vi "Process metadata.vi"(0 "reference in":refnum<class "Force Curve_tdms.lvclass">, 5 "error in (no error)":errorcluster) -> (14 "reference out":refnum<class "Force Curve_tdms.lvclass">, 19 "error out":errorcluster)   [LabVIEW 2019, in "Force Curve_tdms.lvclass"]
uses:
  Force Curve_tdms.lvclass
  TDMS_DataHandler_class/property name combo box.ctl
  Fcurve Meta data analysis.ctl
  TDMS_DataHandler_class/TDMS_DataHandler.lvclass
panel:
  out "Fcurve Raw Metadata.property names":string[](array[string])
  out "Fcurve Raw Metadata.property values":variant[](array[variant])
  out "Array":i32[](array[numeric])
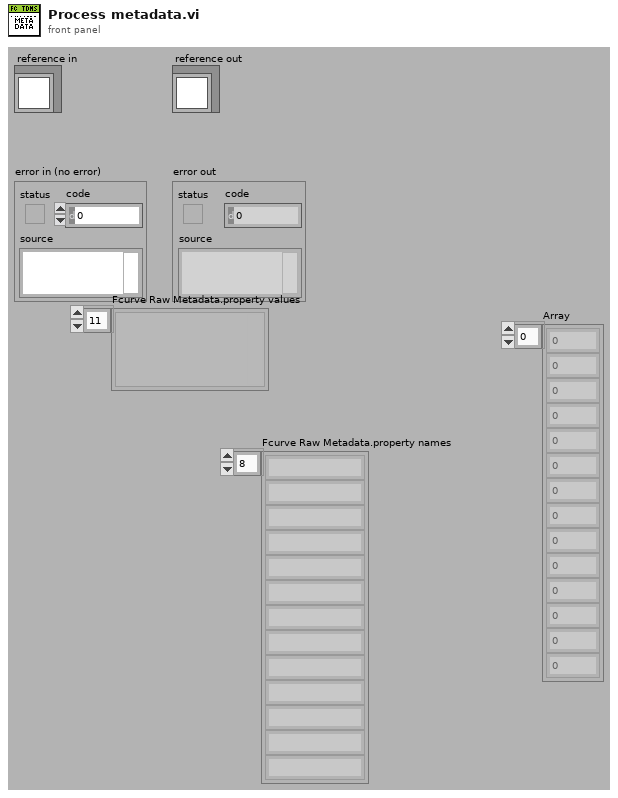
[diagram p1: front panel]
types:
  T1 = typedef "TDMS_DataHandler.lvclass/property name combo box.ctl" = string
  T2 = typedef "Force Curve_tdms.lvclass/Fcurve Meta data analysis.ctl" = cluster{"dt (us)":dbl, "Dec Factor":dbl, "Z piezo Sensitivity (nm/V)":dbl, "K (N/m)":dbl, "Sp (V)":dbl, "Contact (ms)":dbl, "Zpos contact":dbl, "Vel_app (nm/s)":dbl, "Vel_ret (nm/s)":dbl, "deltaV (nm)":dbl, "Def_V0 (v)":dbl, "Decimating Factor":dbl}
  T3 = typedef "Force Curve_tdms.lvclass/ObjectAttributesRef.ctl" = refnum<data-value>
  T4 = typedef "Force Curve_tdms.lvclass/ObjectAttributes.ctl" = cluster{"MyAttribute":dbl, "Processed data":waveform(dbl)[], "Fcurve Raw Metadata":T5, "Fcurve Metadata":T2, "Fcurve index":T6, "Tau Delay (ms)":dbl, "Contact Spread of dev":dbl, "Fcurve":T7}
  T5 = typedef "TDMS_DataHandler.lvclass/Fcurve Meta data.ctl" = cluster{"property names":string[], "property values":variant[]}
  T6 = typedef "Force Curve_tdms.lvclass/Fcurve Index .ctl" = cluster{"Setpoint index":i32, "Max force index":i32, "Contact point index":i32, "Appoach indices":cluster{"Start":i32, "End":i32}, "Contact indices":cluster{"Start":i32, "End":i32}, "Retract indices":cluster{"Start":i32, "End":i32}}
  T7 = typedef "Force Curve_tdms.lvclass/Force Curve data.ctl" = cluster{"Approach":cluster{"X":dbl[], "Y":dbl[]}, "Contact":cluster{"X":dbl[], "Y":dbl[]}, "Retract":cluster{"X":dbl[], "Y":dbl[]}}
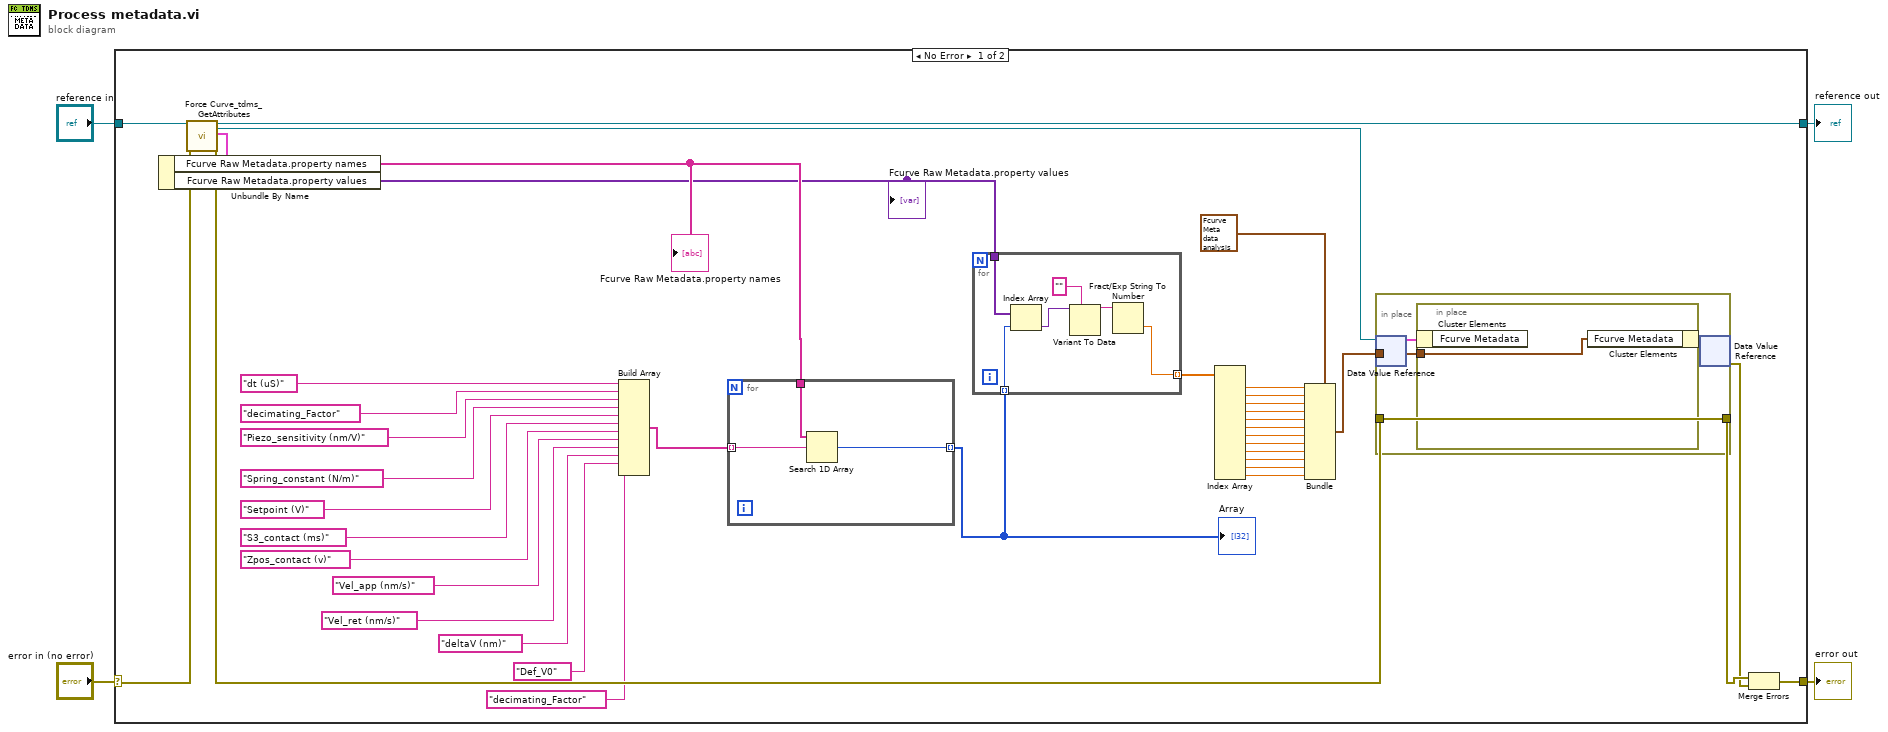
[diagram p0: block diagram]
diagram:
  n1 = case shown="No Error" "error in (no error)" {
    selector: "error in (no error)" -> [w41 w60]
    tunnel: [w44 w60] -> w3
    tunnel: [w42 w59] -> w1
    tunnel: "reference in" -> [w43 w59]
    frame No Error {
      n2 = call "Force Curve_tdms_GetAttributes.vi"("reference in"=w43, "error in (no error)"=w41) -> ("reference out"=w42:refnum<class "Force Curve_tdms.lvclass">, "attributes ref"=w36:T3, "attributes"=w39:T4, "error out"=w40:errorcluster)  [unwired: 14 in]
      n3 = Unbundle By Name(w39) -> ("Fcurve Raw Metadata.property names"=w27:string[], "Fcurve Raw Metadata.property values"=w17:variant[])
      "Fcurve Raw Metadata.property values" <- w17
      "Fcurve Raw Metadata.property names" <- w27
      n4 = Build Array(T1 "dt (uS)" ("Combo Box"), T1 "decimating_Factor" ("Combo Box"), T1 "Piezo_sensitivity (nm/V)" ("Combo Box"), T1 "Spring_constant (N/m)" ("Combo Box"), T1 "Setpoint (V)" ("Combo Box"), T1 "S3_contact (ms)" ("Combo Box"), T1 "Zpos_contact (v)" ("Combo Box"), T1 "Vel_app (nm/s)" ("element"), T1 "Vel_ret (nm/s)" ("element"), T1 "deltaV (nm)" ("element"), T1 "Def_V0" ("element"), T1 "decimating_Factor" ("element")) -> (w28:T1[])
      n5 = for {
        tunnel: w27 -> [w53]
        tunnel: w28 -> [w52] mode=indexing
        tunnel: [w51] -> w15 mode=indexing
        n6 = Search 1D Array(1D array=w53, element=w52) -> (index of element=w51:i32)  [unwired: 1 in]
      }
      "Array" <- w15
      n7 = for {
        tunnel: w17 -> [w50]
        tunnel: [w45] -> w16 mode=indexing
        tunnel: w15 -> [w49] mode=indexing
        n8 = Index Array(array=w50, index=w49) -> (element=w48:variant)
        n9 = Variant To Data(type="", Variant=w48) -> (data=w46:string)  [unwired: 1 in, 1 out]
        n10 = Fract/Exp String To Number(string=w46) -> (number=w45:dbl)  [unwired: 3 in, 1 out]
      }
      n11 = Index Array(array=w16) -> (element #1=w25:dbl, element #2=w24:dbl, element #3=w23:dbl, element #4=w22:dbl, element #5=w21:dbl, element #6=w20:dbl, element #7=w19:dbl, element #8=w10:dbl, element #9=w9:dbl, element #10=w8:dbl, element #11=w7:dbl, element #12=w5:dbl)  [unwired: 12 in]
      n12 = Bundle(cluster=T2 {"dt (us)"=0.0, "Dec Factor"=0.0, "Z piezo Sensitivity (nm/V)"=0.0, "K (N/m)"=0.0, "Sp (V)"=0.0, "Contact (ms)"=0.0, "Zpos contact"=0.0, "Vel_app (nm/s)"=0.0, "Vel_ret (nm/s)"=0.0, "deltaV (nm)"=0.0, "Def_V0 (v)"=0.0, "Decimating Factor"=0.0} ("Fcurve Metadata"), "dt (us)"=w25, "Dec Factor"=w24, "Z piezo Sensitivity (nm/V)"=w23, "K (N/m)"=w22, "Sp (V)"=w21, "Contact (ms)"=w20, "Zpos contact"=w19, "Vel_app (nm/s)"=w10, "Vel_ret (nm/s)"=w9, "deltaV (nm)"=w8, "Def_V0 (v)"=w7, "Decimating Factor"=w5) -> (w18:T2)
      n13 = in-place {
        in-place-border: w40 -> [w55]
        in-place-border: [w55] -> w38
        in-place-border: w18 -> [w54]
        n14 = in-place-dvr #1(w36) -> (w56:T4)  [unwired: 1 out]
        n15 = in-place {
          in-place-border: w54 -> [w58]
          n16 = in-place-cluster #2(w56) -> ()  [unwired: 1 out]
          n17 = in-place-cluster #2("Fcurve Metadata"=w58) -> (w57:T4)
        }
        n18 = in-place-dvr #1(w57) -> (w37:errorcluster)  [unwired: 1 out]
      }
      n19 = Merge Errors(w38, w37) -> (w44:errorcluster)
    }
    frame Error {
    }
  }
  "error out" <- w3
  "reference out" <- w1
